vi "Untitled 1.vi"() -> ()   [LabVIEW 2017]
panel:
  out "vi reference":refnum<vi>
  in  "application reference (local)":refnum<vi>
  in  "vi path":path
  in  "options":i32 format="%.0x"
  in  "type specifier VI Refnum (for type only)":refnum<vi>
  in  "password (\"\")":string
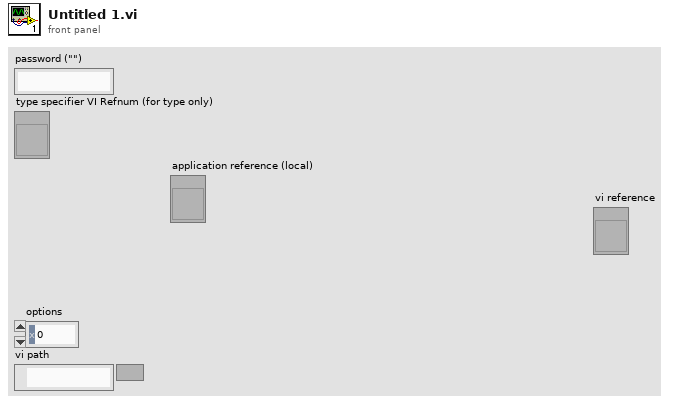
[diagram p1: front panel]
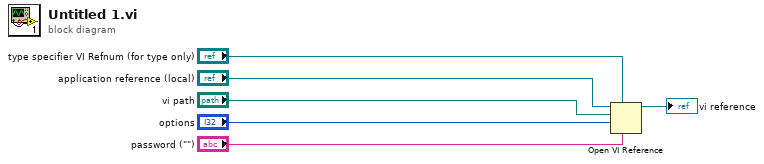
[diagram p0: block diagram]
diagram:
  n1 = Open VI Reference(type specifier VI Refnum (for type only)="type specifier VI Refnum (for type only)", application reference (local)="application reference (local)", vi path="vi path", options="options", password ("")="password (\"\")") -> (vi reference=→"vi reference":refnum<vi>)  [unwired: 1 in, 1 out]
